vi "Receiver_Example - 2 Channel - Experiment_6.vi"() -> ()   [LabVIEW 2022 SP3]
panel:
  out "iterationsIM":dbl
  in  "State":i32
  in  "Counter":dbl
  in  "OFDM - 4QAM/16QAM":bool
  out "Iterations 2":i32
  in  "Tab Control 3":enum32{"OFDM - 4QAM", "16QAM"}(tab)
  in  "Tab Control":enum32{"USRP Parameters", "Rx Info", "BER"}(tab)
  in  "USRP ControledParameters":T1={"Active Antenna"="RX2", "Gain (dB)"=10.0, "Carrier Frequency"=2400000000.0, "IQ Rate"=2000000.0, "Active channels"="0,1"} {"IQ Rate" format="%#_6p"; "Carrier Frequency" format="%#_6p"; "Gain (dB)" format="%#_6f"}
  in  "Device selection":refnum<k15>="RIO0"
  in  "Trigger level":dbl=0.005 format="%f"
  out "CH0":T2
  out "CH1":T2
  out "SIG valid? - CH1":bool
  out "SIG valid? - CH0":bool
  out "Frequency offset - CH1":dbl
  out "Frequency offset - CH0":dbl
  out "Coerced Parameters":T3={"IQ Rate"=100000.0, "Carrier  Freq."=100000.0, "Gain"=0.0} {"Gain" format="%#_6f"; "Carrier  Freq." format="%#_6p"; "IQ Rate" format="%#_6p"}
  out "Error out":errorcluster
  in  "Expected message LP - CH0":string="Non Critical Data\nNon Critical Data\nNon Critical Data\nNon Critical Data\nNon Critical Data"
  in  "Expected message - CH1":string="Critical Dataaaaa\nCritical Dataaaaa\nCritical Dataaaaa\nCritical Dataaaaa\nCritical Dataaaaa"
  out "Expected message LP Detected CH0":string="Non Critical Data\nNon Critical Data\nNon Critical Data\nNon Critical Data\nNon Critical Data"
  out "Expected message HP Detected CH1":string="Non Critical Data\nNon Critical Data\nNon Critical Data\nNon Critical Data\nNon Critical Data"
  in  "Boolean":bool
  in  "Boolean 3":bool
  out "Expected message HP Detected CH0":string="Non Critical Data\nNon Critical Data\nNon Critical Data\nNon Critical Data\nNon Critical Data"
  in  "Expected message HP - CH0":string="Critical Dataaaaa\nCritical Dataaaaa\nCritical Dataaaaa\nCritical Dataaaaa\nCritical Dataaaaa"
  in  "Boolean 2":bool
  out "Inst. BER HP - CH0":dbl format="%#_4g"
  out "Acc. BER HP - CH0":dbl format="%#_4g"
  out "Acum. Err HP - CH0":dbl
  out "No. Bits HP - CH0":dbl
  out "Acc. BER LP - CH0":dbl format="%#_4g"
  out "Inst. BER - CH1":dbl format="%#_4g"
  out "Inst. BER LP - CH0":dbl format="%#_4g"
  out "No. Bits - CH1":dbl
  out "No. Bits LP - CH0":dbl
  out "Acum. Err - CH1":dbl
  out "Acum. Err LP - CH0":dbl
  in  "Record BER":bool
  in  "Refresh Button":bool
  out "Acc. BER - CH1":dbl format="%#_4g"
  in  "Low-Power Window Size - CH0":dbl=15.0 format="%#_6p"
  in  "High-Power Window Size":dbl=15.0 format="%#_6p"
  out "High-Power Image 2":T4(plugin-control)
  in  "Tab Control 2":enum32{"1 Channel", "2 Channel"}(tab)
  out "Constellation Map 1 Channel":cdb[](graph)
  out "Low-Power BER - 1 Channel":dbl(graph)
  out "High-Power BER - 1 Channel":dbl(graph)
  out "High-Power Decoded message - 1 Channel":string
  out "Low-Power Decoded message - 1 Channel":string
  out "Low-Power Decoded message - CH0":string
  out "Decoded message - CH1":string
  out "Constellation Map 2 Channel":cluster{"Constellation":cdb[]}[](graph)
  out "Low-Power BER - CH0":dbl(graph)
  out "High-Power BER":T5(graph)
  out "High-Power Decoded message - CH0":string
  out "CH1 2":bool
  out "CH0 2":bool
  in  "Channel":bool
  out "Reconstructed Image":T4(plugin-control)
  out "Expected message  HP  Detected 2":string="Critical Dataaaaa\nCritical Dataaaaa\nCritical Dataaaaa\nCritical Dataaaaa\nCritical Dataaaaa"
  in  "Boolean 4":bool
  in  "High-Power Window Size 2":dbl=15.0 format="%#_6p"
  out "High-Power Instantaneous BER Graph 2":u8(slide) scale=0.0..100.0
  out "High-Power BER Graph 2":dbl(graph)
  out "No. Bits HP 2":dbl
  out "Acc. BER  HP 2":dbl format="%#_4g"
  out "Acum. Err HP 2":dbl
  out "Inst. BER HP 2":dbl format="%#_4g"
  in  "Expected message 2 HP 2":string="Critical Dataaaaa\nCritical Dataaaaa\nCritical Dataaaaa\nCritical Dataaaaa\nCritical Dataaaaa"
  out "High-Power Decoded Message 2":string
  in  "Record BER 2":bool
  out "Constellation Map 2":cdb[](graph)
  out "Frequency offset 2":dbl
  out "SIG valid? 2":bool
  in  "Refresh Button 2":bool
  out "Error out 2":errorcluster
  in  "error in (no error)":errorcluster
  # "OFDM Superposition Coded Receiver"
  # "1 Channel"
  # "2 Channel"
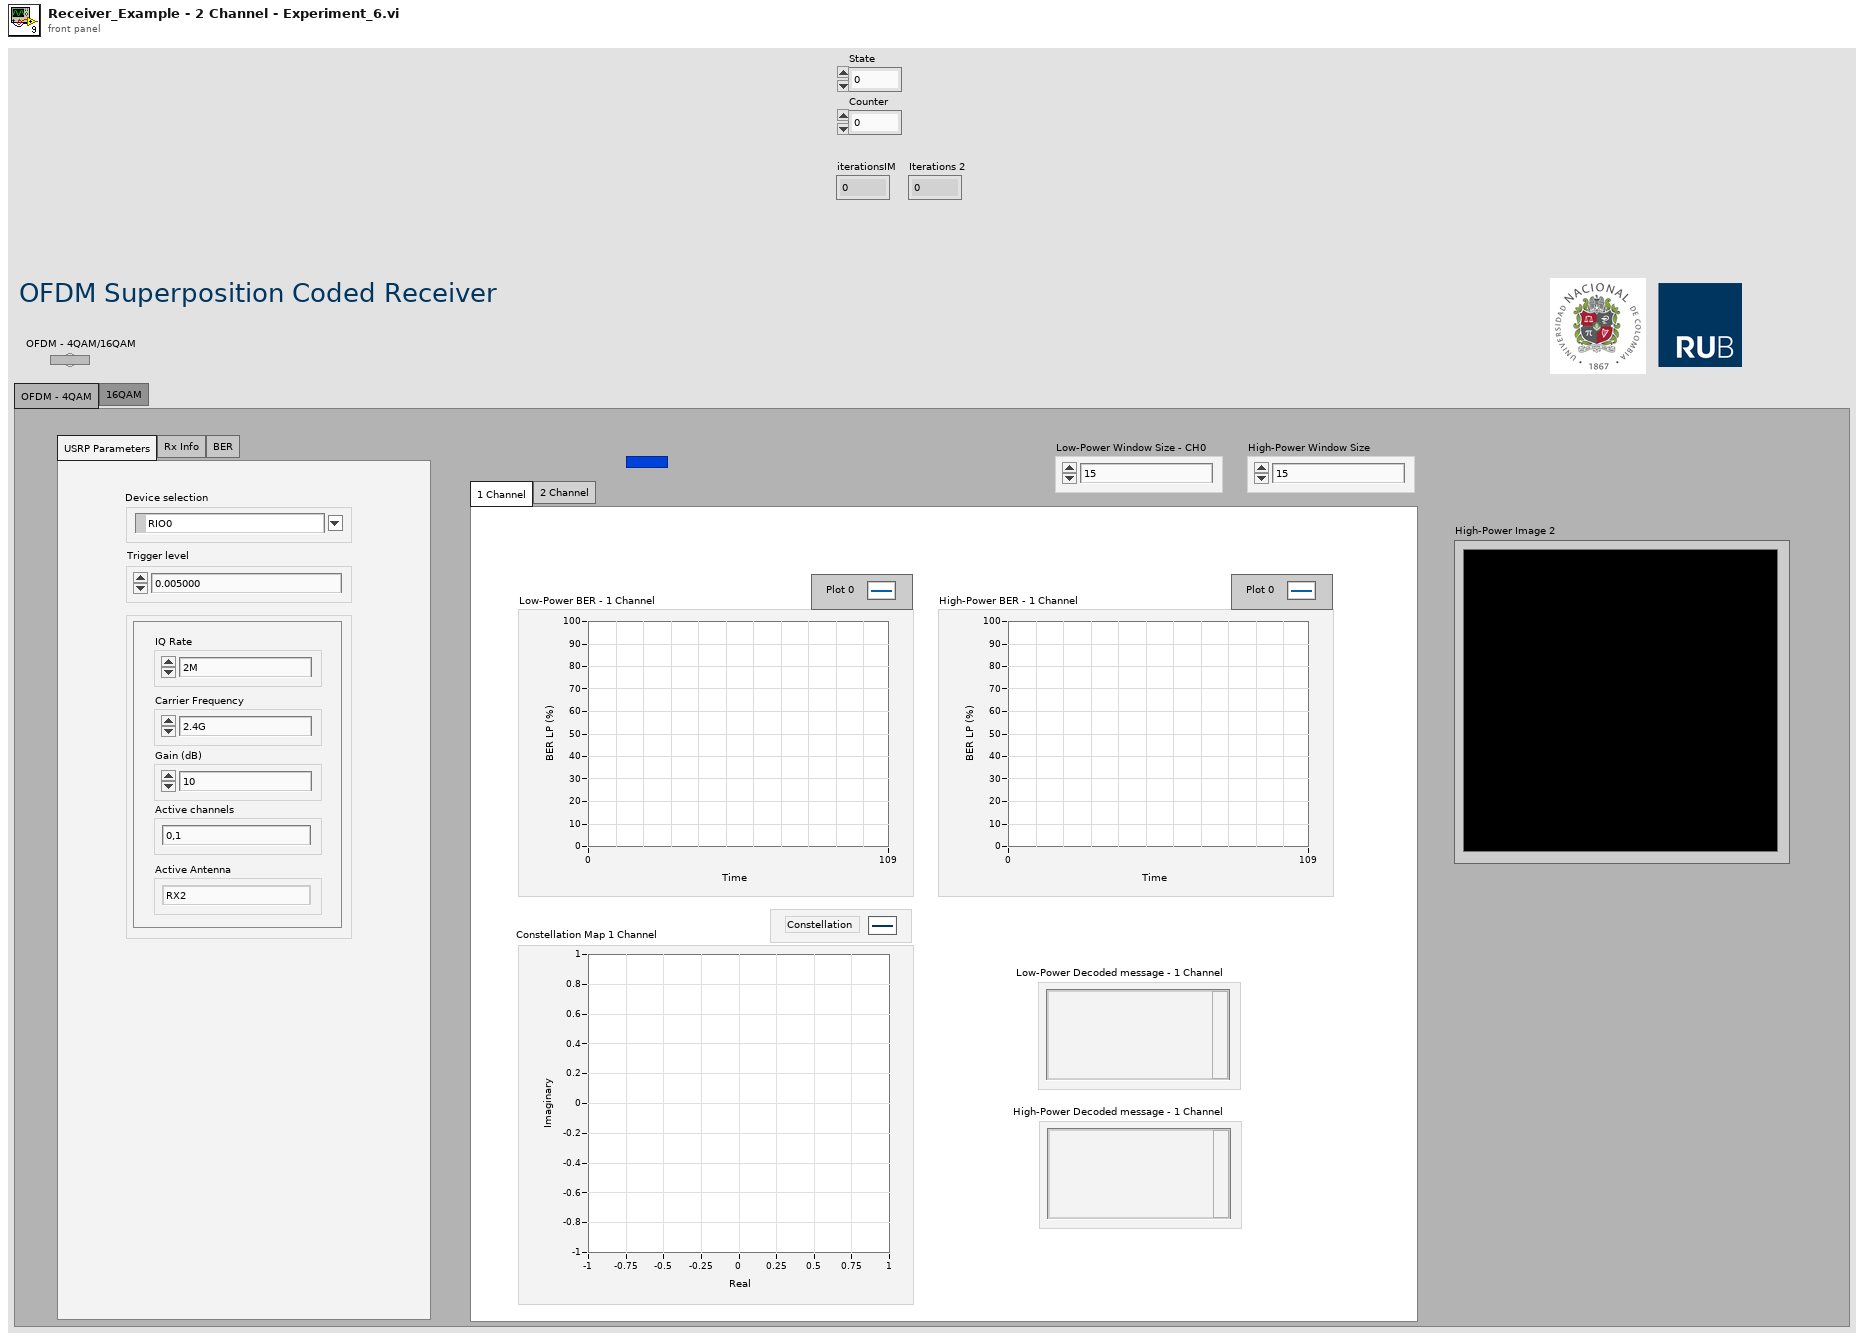
[diagram p1: front panel]
types:
  T1 = cluster{"Active Antenna":string, "Gain (dB)":dbl, "Carrier Frequency":dbl, "IQ Rate":dbl, "Active channels":string}
  T2 = cluster{"Modulation type":enum16{"QPSK(4QAM)", "64QAM", "16QAM", "BPSK"}, "BCC rate (k/n)":enum16{"1/2", "2/3", "3/4"}}
  T3 = cluster{"IQ Rate":dbl, "Carrier  Freq.":dbl, "Gain":dbl}
  T4 = typedef "IMAQ Image.ctl" = refnum<image>
  T5 = cluster{"Graph Instantaneous BER":dbl, "Graph Instantaneous BER":dbl, "Inst. BER - CH1":dbl}
  T6 = cluster{"coerced IQ rate":dbl, "coerced carrier frequency":dbl, "coerced gain":dbl}
  T7 = cluster{"Graph Instantaneous BER":dbl, "Graph Instantaneous BER":dbl, "Graph Instantaneous BER":dbl}
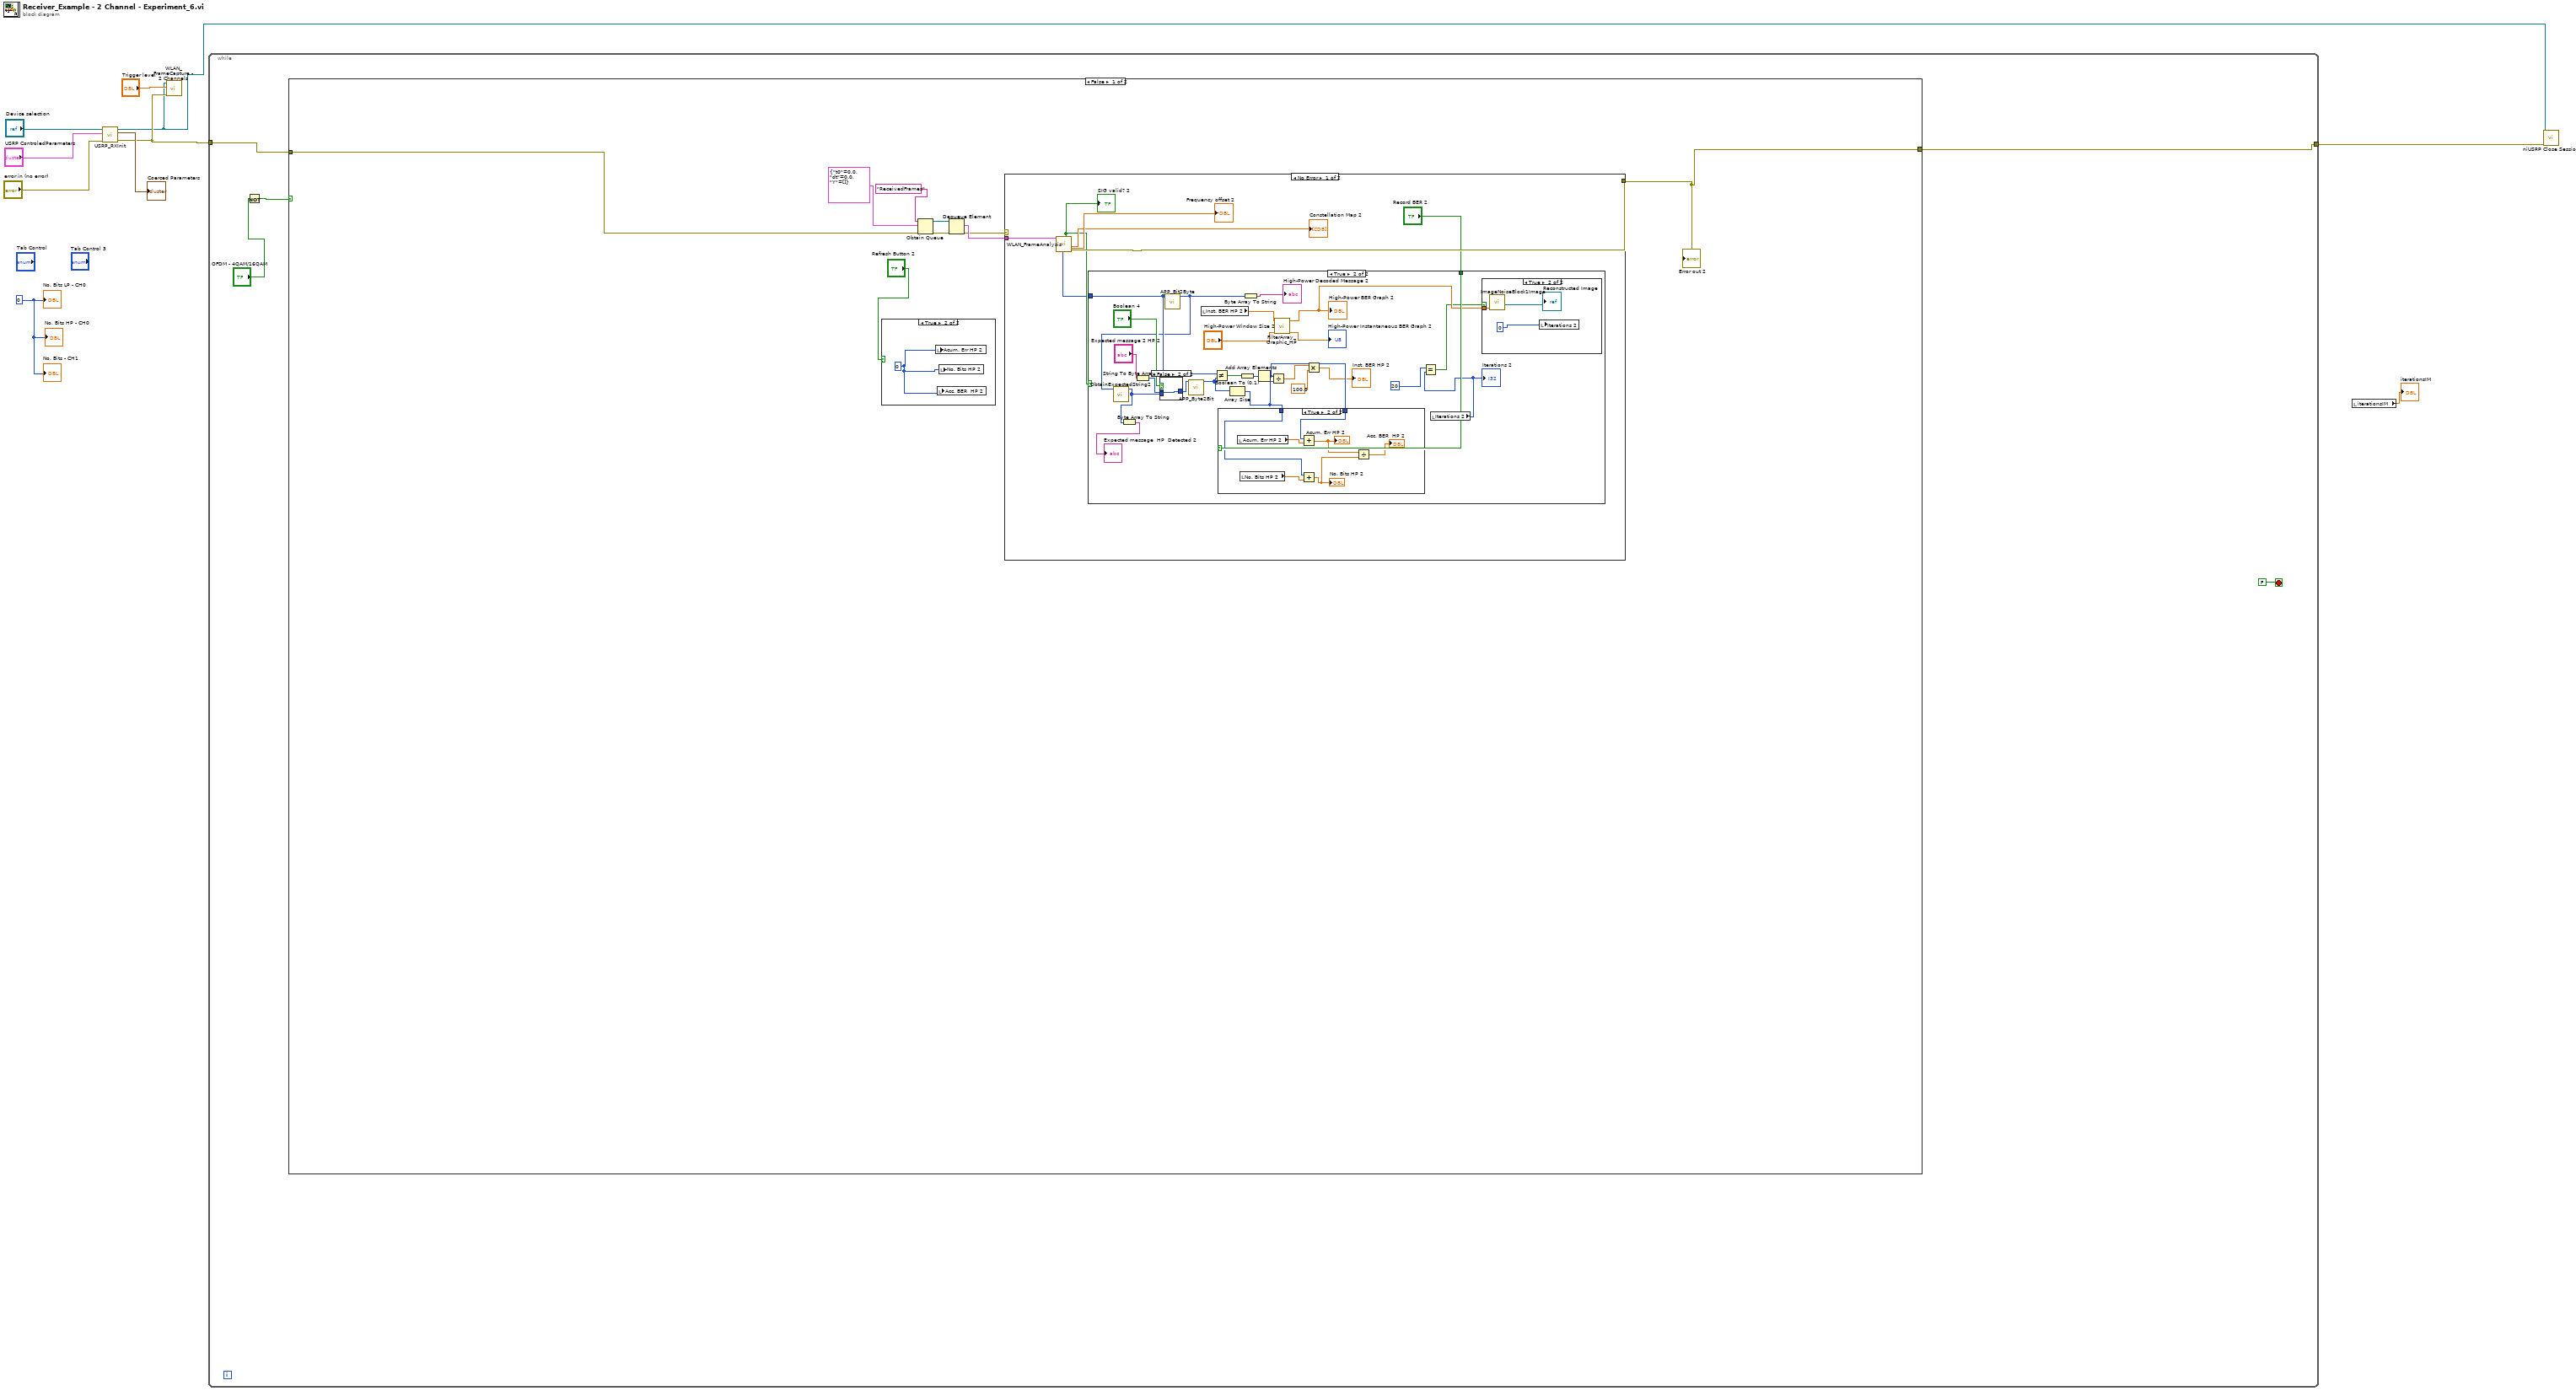
[diagram p0: block diagram]
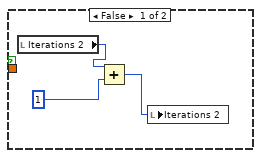
[diagram p4: hidden frame]
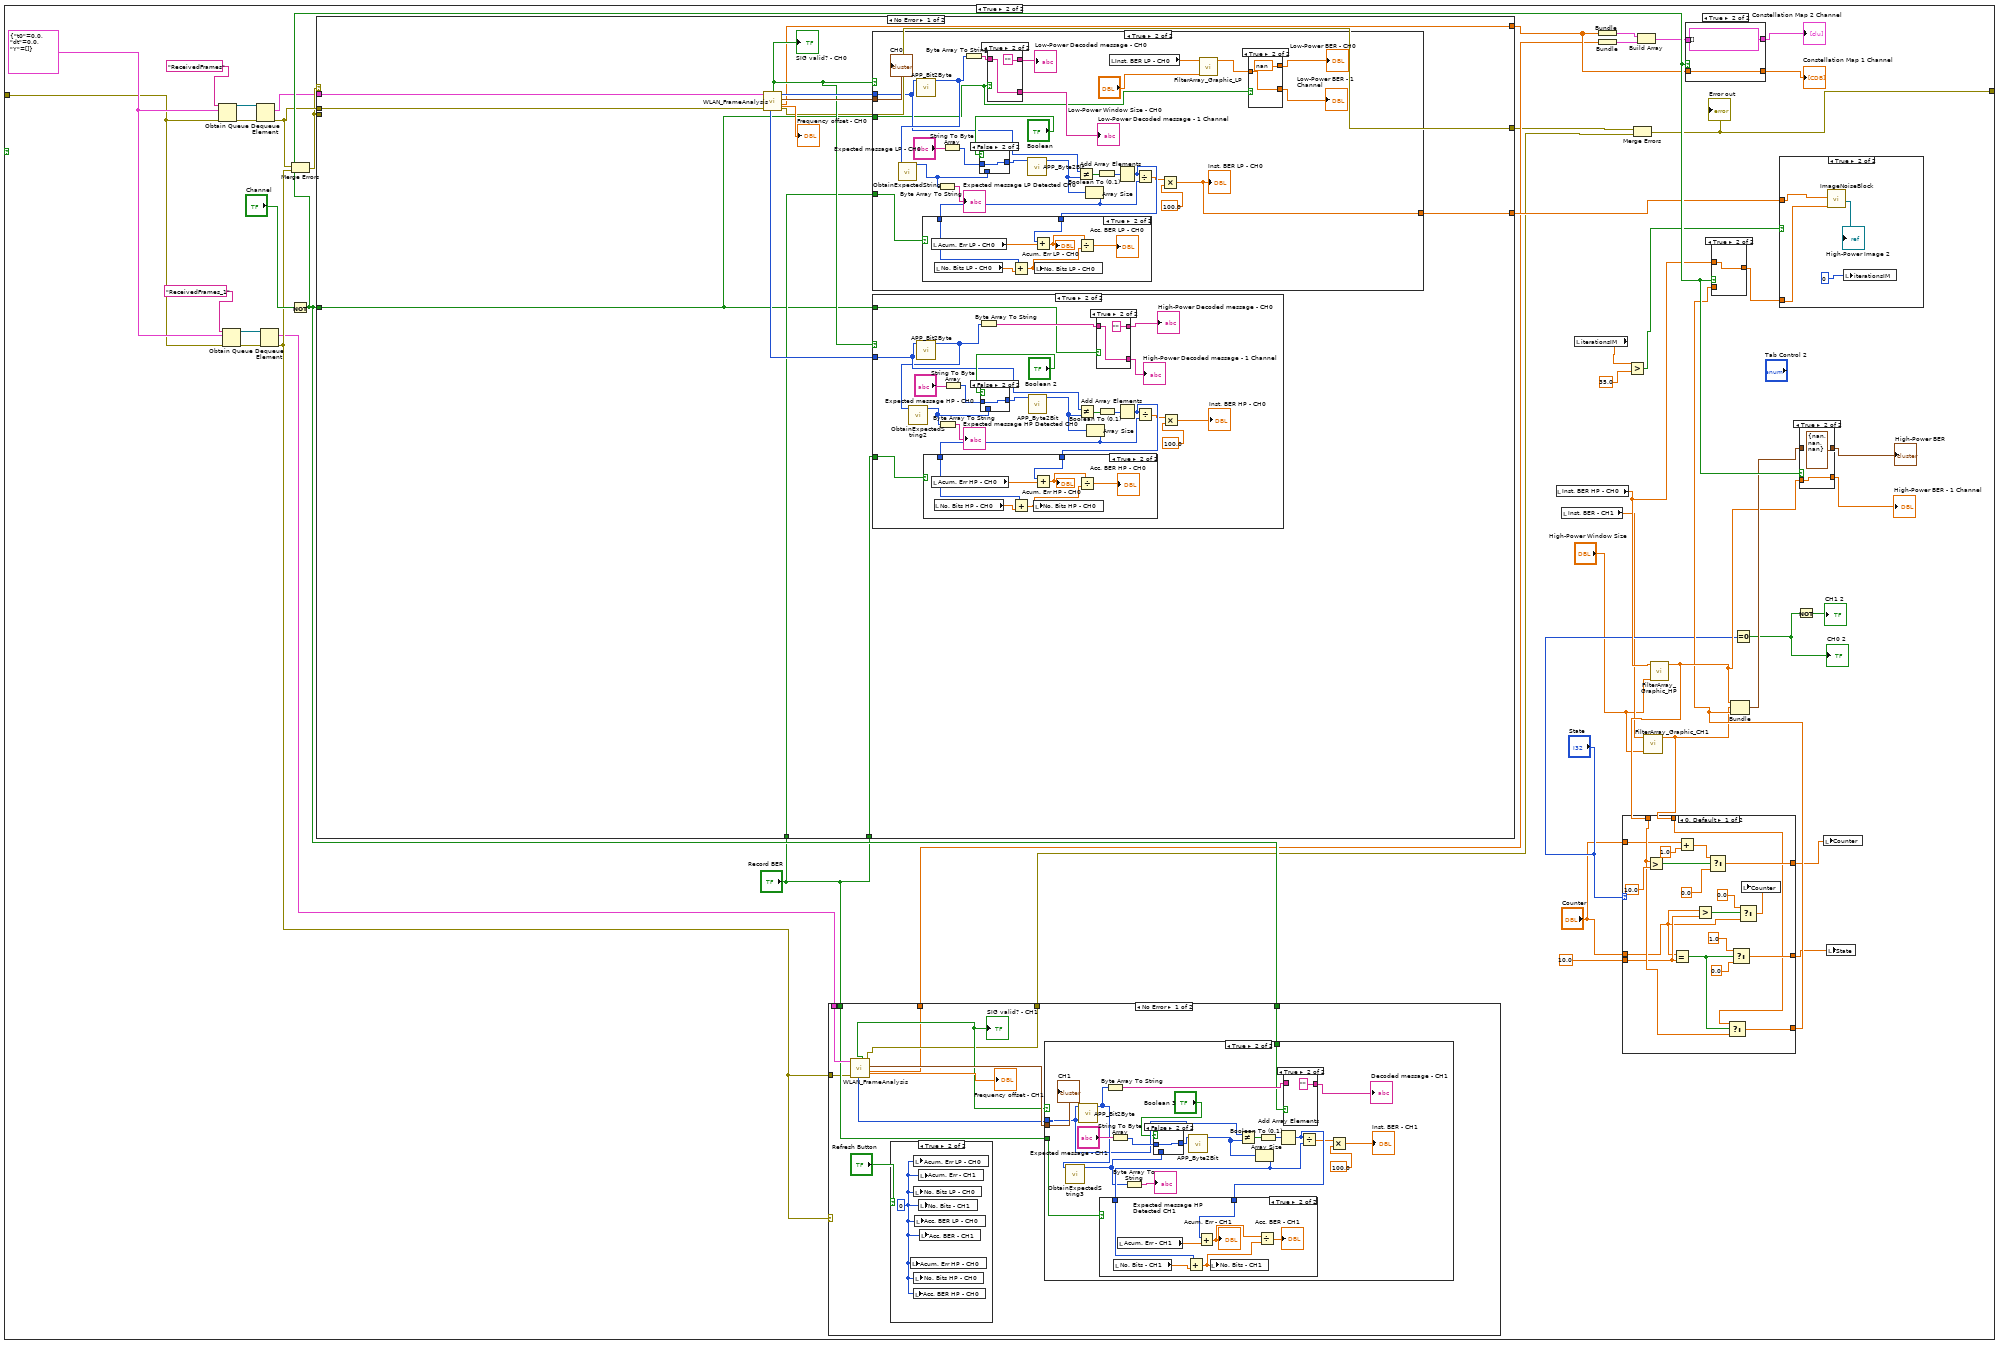
[diagram p8: hidden frame]
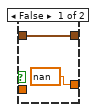
[diagram p9: hidden frame]
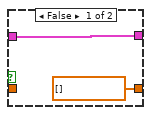
[diagram p11: hidden frame]
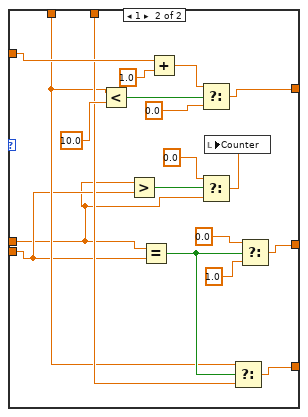
[diagram p12: hidden frame]
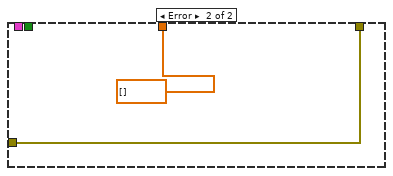
[diagram p18: hidden frame]
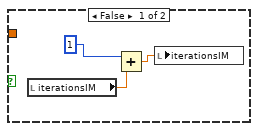
[diagram p19: hidden frame]
diagram:
  w2 = 0
  n1 = call "USRP_RXInit.vi"("device names"="Device selection", "USRP ControledParameters"="USRP ControledParameters", "error in (no error)"="error in (no error)") -> ("session handle out"=w5:refnum<k15>, "USRP CoercedParamters"=→"Coerced Parameters":T6, "error out"=w8:errorcluster)  [unwired: 5 in]
  n2 = call "WLAN_FrameCapture - 2 Channels.vi"("error in (no error)"=w8, "Trigger level"="Trigger level", "session handle"=w5) -> ()  [unwired: 8 in]
  n3 = while {
    tunnel: w8 -> [w15]
    tunnel: [w14] -> w6
    stop <- FALSE stop-if-true
    n4 = Not(x="OFDM - 4QAM/16QAM") -> (.not. x?=w12:bool)
    n5 = case shown="False" w12 {
      tunnel: w15 -> [w17 w75]
      tunnel: [w16 w74] -> w14
      frame False {
        n6 = case shown="True" "Refresh Button 2" {
          frame False {
          }
          frame True {
            w25 = 0
            n7 = local write "Acum. Err HP 2"(w25) -> ()
            n8 = local write "Acc. BER  HP 2"(w25) -> ()
            n9 = local write "No. Bits HP 2"(w25) -> ()
          }
        }
        n10 = Obtain Queue(name (unnamed)="ReceivedFrames", element data type=cluster{"t0":dbl, "dt":dbl, "Y":cdb[]} {"t0"=0.0, "dt"=0.0, "Y"=[]} ("data"), error in (no error)=w17) -> (queue out=w18:refnum<queue>, error out=w21:errorcluster)  [unwired: 2 in, 1 out]
        n11 = Dequeue Element(queue=w18, error in (no error)=w21) -> (element=w20:cluster{"t0":dbl, "dt":dbl, "Y":cdb[]}, error out=w19:errorcluster)  [unwired: 1 in, 2 out]
        n12 = case shown="No Error" w19 {
          selector: w19 -> [_ w73]
          tunnel: w20 -> [w31 _]
          tunnel: [w32 w73] -> w16
          frame No Error {
            n13 = call "WLAN_FrameAnalysis.vi"("input cluster"=w31) -> ("error out"=w32:errorcluster, "Constellation"=→"Constellation Map 2":cdb[], "Frequency offset"=→"Frequency offset 2":dbl, "SIG valid?"=w27:bool, "outputbitsHP"=w26:i8[])  [unwired: 4 in, 2 out]
            "SIG valid? 2" <- w27
            n14 = case shown="True" w27 {
              tunnel: "Record BER 2" -> [_ w51]
              tunnel: w26 -> [_ w46]
              frame False {
              }
              frame True {
                n15 = String To Byte Array(string="Expected message 2 HP 2") -> (unsigned byte array=w44:u8[])
                n16 = call "APP_Bit2Byte.vi"("input bit stream"=w46) -> ("output byte stream"=w40:u8[])  [unwired: 10 in]
                n17 = call "ObtainExpectedString2.vi"("Array"=w40) -> ("detectedMessage"=w42:i8[])  [unwired: 9 in]
                n18 = Byte Array To String(unsigned byte array=w42) -> (string=→"Expected message  HP  Detected 2":string)
                n19 = case shown="False" "Boolean 4" {
                  tunnel: [w64 w65] -> w45
                  tunnel: w44 -> [_ w65]
                  tunnel: w42 -> [w64 _]
                  frame True {
                  }
                  frame False {
                  }
                }
                n20 = call "APP_Byte2Bit.vi"("input byte stream"=w45) -> ("output bit stream"=w47:i8[])  [unwired: 10 in]
                n21 = local read "Inst. BER HP 2"() -> (w50:dbl)
                n22 = Not Equal?(x=w46, y=w47) -> (x != y?=w55:bool[])
                n23 = Array Size(array=w47) -> (size(s)=w52:i32)
                n24 = Boolean To (0,1)(Boolean=w55) -> (0, 1=w54:i16[])
                n25 = Byte Array To String(unsigned byte array=w40) -> (string=→"High-Power Decoded Message 2":string)
                n26 = Add Array Elements(numeric array=w54) -> (sum=w53:i16)
                n27 = case shown="True" w51 {
                  tunnel: w53 -> [_ w71]
                  tunnel: w52 -> [_ w66]
                  frame False {
                  }
                  frame True {
                    n28 = local read "Acum. Err HP 2"() -> (w72:dbl)
                    n29 = local read "No. Bits HP 2"() -> (w68:dbl)
                    n30 = Add(x=w71, y=w72) -> (x+y=w70:dbl)
                    "Acum. Err HP 2" <- w70
                    n31 = Add(x=w66, y=w68) -> (x+y=w67:dbl)
                    "No. Bits HP 2" <- w67
                    n32 = Divide(x=w70, y=w67) -> (x/y=→"Acc. BER  HP 2":dbl)
                  }
                }
                n33 = Divide(x=w53, y=w52) -> (x/y=w39:dbl)
                n34 = call "FilterArray_Graphic_HP.vi"("Window Size"="High-Power Window Size 2", "Instantaneous BER"=w50) -> ("Slide Bar"=→"High-Power Instantaneous BER Graph 2":dbl, "Graph Instantaneous BER"=w36:dbl)  [unwired: 4 in]
                "High-Power BER Graph 2" <- w36
                n35 = Multiply(x=w39, y=100.0) -> (x*y=→"Inst. BER HP 2":dbl)
                n36 = local read "Iterations 2"() -> (w34:i32)
                "Iterations 2" <- w34
                n37 = Equal?(x=20, y=w34) -> (x = y?=w33:bool)
                n38 = case shown="True" w33 {
                  tunnel: w36 -> [_ w63]
                  frame False {
                    n39 = local read "Iterations 2"() -> (w60:i32)
                    n40 = Add(x=w60, y=1) -> (x+y=w58:i32)
                    n41 = local write "Iterations 2"(w58) -> ()
                  }
                  frame True {
                    n42 = call "ImageNoiseBlock1Image.vi"("BERHP"=w63) -> ("High-Power Image"=→"Reconstructed Image":T4)  [unwired: 9 in]
                    n43 = local write "Iterations 2"(0) -> ()
                  }
                }
              }
            }
          }
          frame Error {
          }
        }
        "Error out 2" <- w16
      }
      frame True {
        w120 = cluster{"t0":dbl, "dt":dbl, "Y":cdb[]} {"t0"=0.0, "dt"=0.0, "Y"=[]} ("data")
        n44 = Obtain Queue(name (unnamed)="ReceivedFrames", element data type=w120, error in (no error)=w75) -> (queue out=w76:refnum<queue>, error out=w78:errorcluster)  [unwired: 2 in, 1 out]
        n45 = Obtain Queue(name (unnamed)="ReceivedFrames_1", element data type=w120, error in (no error)=w75) -> (queue out=w80:refnum<queue>, error out=w81:errorcluster)  [unwired: 2 in, 1 out]
        n46 = Dequeue Element(queue=w76, error in (no error)=w78) -> (element=w77:cluster{"t0":dbl, "dt":dbl, "Y":cdb[]}, error out=w84:errorcluster)  [unwired: 1 in, 2 out]
        n47 = Dequeue Element(queue=w80, error in (no error)=w81) -> (element=w89:cluster{"t0":dbl, "dt":dbl, "Y":cdb[]}, error out=w93:errorcluster)  [unwired: 1 in, 2 out]
        n48 = Not(x="Channel") -> (.not. x?=w119:bool)
        n49 = Merge Errors(w84, w93) -> (w83:errorcluster)
        n50 = case shown="No Error" w83 {
          tunnel: w77 -> [w231 _]
          tunnel: w83 -> [_ w315]
          tunnel: w84 -> [w228 _]
          tunnel: [w227 100] -> w95
          tunnel: [w226 dbl[] []] -> w107
          tunnel: [w225 w315] -> w90
          tunnel: "Record BER" -> [w224 _]
          tunnel: "Record BER" -> [w223 _]
          tunnel: w119 -> [w222 _]
          frame No Error {
            n51 = call "WLAN_FrameAnalysis.vi"("error in (no error)"=w228, "input cluster"=w231) -> ("error out"=w225:errorcluster, "Constellation"=w226:cdb[], "Modulation parameter"=w232:T2, "output bits"=w233:i8[], "Frequency offset"=→"Frequency offset - CH0":dbl, "SIG valid?"=w229:bool, "outputbitsHP"=w230:i8[])  [unwired: 3 in]
            "SIG valid? - CH0" <- w229
            n52 = case shown="True" w229 {
              tunnel: w233 -> [_ w278]
              tunnel: w232 -> [_ w296]
              tunnel: w223 -> [_ w292]
              tunnel: [100.0 w277] -> w227
              tunnel: w222 -> [_ w270]
              frame False {
              }
              frame True {
                n53 = call "APP_Bit2Byte.vi"("input bit stream"=w278) -> ("output byte stream"=w282:u8[])  [unwired: 10 in]
                n54 = call "ObtainExpectedString.vi"("Array"=w282) -> ("detectedMessage"=w279:i8[])  [unwired: 9 in]
                n55 = Byte Array To String(unsigned byte array=w279) -> (string=→"Expected message LP Detected CH0":string)
                n56 = String To Byte Array(string="Expected message LP - CH0") -> (unsigned byte array=w283:u8[])
                n57 = Byte Array To String(unsigned byte array=w282) -> (string=w276:string)
                n58 = case shown="False" "Boolean" {
                  tunnel: [w305 w306] -> w285
                  tunnel: w283 -> [_ w306]
                  tunnel: w279 -> [w305 _]
                  frame True {
                  }
                  frame False {
                  }
                }
                n59 = case shown="True" w270 {
                  tunnel: w276 -> [w302 w304]
                  tunnel: ["" ("string") w304] -> w275
                  tunnel: [w302 "" ("string")] -> w274
                  frame False {
                  }
                  frame True {
                  }
                }
                "Low-Power Decoded message - CH0" <- w274
                "Low-Power Decoded message - 1 Channel" <- w275
                n60 = call "APP_Byte2Bit.vi"("input byte stream"=w285) -> ("output bit stream"=w284:i8[])  [unwired: 10 in]
                n61 = Not Equal?(x=w278, y=w284) -> (x != y?=w294:bool[])
                n62 = Array Size(array=w284) -> (size(s)=w291:i32)
                n63 = Boolean To (0,1)(Boolean=w294) -> (0, 1=w295:i16[])
                n64 = local read "Inst. BER LP - CH0"() -> (w288:dbl)
                n65 = Add Array Elements(numeric array=w295) -> (sum=w290:i16)
                n66 = case shown="True" w292 {
                  tunnel: w291 -> [_ w312]
                  tunnel: w290 -> [_ w310]
                  frame False {
                  }
                  frame True {
                    n67 = local read "Acum. Err LP - CH0"() -> (w311:dbl)
                    n68 = local read "No. Bits LP - CH0"() -> (w313:dbl)
                    n69 = Add(x=w312, y=w313) -> (x+y=w309:dbl)
                    n70 = Add(x=w310, y=w311) -> (x+y=w308:dbl)
                    "Acum. Err LP - CH0" <- w308
                    n71 = local write "No. Bits LP - CH0"(w309) -> ()
                    n72 = Divide(x=w308, y=w309) -> (x/y=→"Acc. BER LP - CH0":dbl)
                  }
                }
                n73 = Divide(x=w290, y=w291) -> (x/y=w287:dbl)
                n74 = Multiply(x=w287, y=100.0) -> (x*y=w277:dbl)
                "Inst. BER LP - CH0" <- w277
                n75 = call "FilterArray_Graphic_LP.vi"("Window Size"="Low-Power Window Size - CH0", "Instantaneous BER"=w288) -> ("Graph Instantaneous BER"=w273:dbl)  [unwired: 4 in, 1 out]
                n76 = case shown="True" w270 {
                  tunnel: w273 -> [w298 w300]
                  tunnel: [nan ("Graph Instantaneous BER") w300] -> w272
                  tunnel: [w298 nan ("Graph Instantaneous BER")] -> w271
                  frame False {
                  }
                  frame True {
                  }
                }
                "Low-Power BER - CH0" <- w271
                "Low-Power BER - 1 Channel" <- w272
                "CH0" <- w296
              }
            }
            n77 = case shown="True" w229 {
              tunnel: w230 -> [_ w242]
              tunnel: w224 -> [_ w252]
              tunnel: w222 -> [_ w235]
              frame False {
              }
              frame True {
                n78 = call "APP_Bit2Byte.vi"("input bit stream"=w242) -> ("output byte stream"=w241:u8[])  [unwired: 10 in]
                n79 = call "ObtainExpectedString2.vi"("Array"=w241) -> ("detectedMessage"=w240:i8[])  [unwired: 9 in]
                n80 = Byte Array To String(unsigned byte array=w240) -> (string=→"Expected message HP Detected CH0":string)
                n81 = String To Byte Array(string="Expected message HP - CH0") -> (unsigned byte array=w245:u8[])
                n82 = Byte Array To String(unsigned byte array=w241) -> (string=w236:string)
                n83 = case shown="False" "Boolean 2" {
                  tunnel: [w260 w261] -> w247
                  tunnel: w245 -> [_ w261]
                  tunnel: w240 -> [w260 _]
                  frame True {
                  }
                  frame False {
                  }
                }
                n84 = call "APP_Byte2Bit.vi"("input byte stream"=w247) -> ("output bit stream"=w246:i8[])  [unwired: 10 in]
                n85 = Not Equal?(x=w242, y=w246) -> (x != y?=w254:bool[])
                n86 = Array Size(array=w246) -> (size(s)=w251:i32)
                n87 = case shown="True" w235 {
                  tunnel: w236 -> [w257 w259]
                  tunnel: ["" ("string") w259] -> w237
                  tunnel: [w257 "" ("string")] -> w238
                  frame False {
                  }
                  frame True {
                  }
                }
                "High-Power Decoded message - CH0" <- w238
                "High-Power Decoded message - 1 Channel" <- w237
                n88 = Boolean To (0,1)(Boolean=w254) -> (0, 1=w255:i16[])
                n89 = Add Array Elements(numeric array=w255) -> (sum=w250:i16)
                n90 = case shown="True" w252 {
                  tunnel: w251 -> [_ w267]
                  tunnel: w250 -> [_ w265]
                  frame False {
                  }
                  frame True {
                    n91 = local read "Acum. Err HP - CH0"() -> (w266:dbl)
                    n92 = local read "No. Bits HP - CH0"() -> (w268:dbl)
                    n93 = Add(x=w267, y=w268) -> (x+y=w264:dbl)
                    n94 = local write "No. Bits HP - CH0"(w264) -> ()
                    n95 = Add(x=w265, y=w266) -> (x+y=w263:dbl)
                    "Acum. Err HP - CH0" <- w263
                    n96 = Divide(x=w263, y=w264) -> (x/y=→"Acc. BER HP - CH0":dbl)
                  }
                }
                n97 = Divide(x=w250, y=w251) -> (x/y=w249:dbl)
                n98 = Multiply(x=w249, y=100.0) -> (x*y=→"Inst. BER HP - CH0":dbl)
              }
            }
          }
          frame Error {
            (unwired) 100
          }
        }
        n99 = case shown="No Error" w93 {
          tunnel: w89 -> [w175 _]
          tunnel: "Record BER" -> [w173 _]
          tunnel: [w172 w214] -> w91
          tunnel: [w171 dbl[] []] -> w92
          tunnel: w93 -> [w170 w214]
          tunnel: w119 -> [w169 _]
          frame No Error {
            n100 = call "WLAN_FrameAnalysis.vi"("error in (no error)"=w170, "input cluster"=w175) -> ("error out"=w172:errorcluster, "Constellation"=w171:cdb[], "Modulation parameter"=w178:T2, "Frequency offset"=→"Frequency offset - CH1":dbl, "SIG valid?"=w174:bool, "outputbitsHP"=w176:i8[])  [unwired: 3 in, 1 out]
            "SIG valid? - CH1" <- w174
            n101 = case shown="True" "Refresh Button" {
              frame False {
              }
              frame True {
                w180 = 0
                n102 = local write "Acum. Err HP - CH0"(w180) -> ()
                n103 = local write "Acc. BER HP - CH0"(w180) -> ()
                n104 = local write "Acum. Err LP - CH0"(w180) -> ()
                n105 = local write "No. Bits LP - CH0"(w180) -> ()
                n106 = local write "No. Bits HP - CH0"(w180) -> ()
                n107 = local write "Acc. BER LP - CH0"(w180) -> ()
                n108 = local write "Acum. Err - CH1"(w180) -> ()
                n109 = local write "No. Bits - CH1"(w180) -> ()
                n110 = local write "Acc. BER - CH1"(w180) -> ()
              }
            }
            n111 = case shown="True" w174 {
              tunnel: w176 -> [_ w187]
              tunnel: w178 -> [_ w201]
              tunnel: w173 -> [_ w184]
              tunnel: w169 -> [_ w181]
              frame False {
              }
              frame True {
                n112 = call "APP_Bit2Byte.vi"("input bit stream"=w187) -> ("output byte stream"=w190:u8[])  [unwired: 10 in]
                n113 = call "ObtainExpectedString3.vi"("Array"=w190) -> ("detectedMessage"=w189:i8[])  [unwired: 9 in]
                n114 = Byte Array To String(unsigned byte array=w190) -> (string=w182:string)
                n115 = String To Byte Array(string="Expected message - CH1") -> (unsigned byte array=w191:u8[])
                n116 = Byte Array To String(unsigned byte array=w189) -> (string=→"Expected message HP Detected CH1":string)
                n117 = case shown="False" "Boolean 3" {
                  tunnel: [w204 w205] -> w193
                  tunnel: w191 -> [_ w205]
                  tunnel: w189 -> [w204 _]
                  frame True {
                  }
                  frame False {
                  }
                }
                n118 = call "APP_Byte2Bit.vi"("input byte stream"=w193) -> ("output bit stream"=w192:i8[])  [unwired: 10 in]
                n119 = Not Equal?(x=w187, y=w192) -> (x != y?=w199:bool[])
                n120 = Array Size(array=w192) -> (size(s)=w197:i32)
                n121 = Boolean To (0,1)(Boolean=w199) -> (0, 1=w200:i16[])
                n122 = Add Array Elements(numeric array=w200) -> (sum=w196:i16)
                n123 = case shown="True" w184 {
                  tunnel: w197 -> [_ w211]
                  tunnel: w196 -> [_ w209]
                  frame False {
                  }
                  frame True {
                    n124 = local read "No. Bits - CH1"() -> (w212:dbl)
                    n125 = local read "Acum. Err - CH1"() -> (w210:dbl)
                    n126 = Add(x=w211, y=w212) -> (x+y=w208:dbl)
                    n127 = Add(x=w209, y=w210) -> (x+y=w207:dbl)
                    "Acum. Err - CH1" <- w207
                    n128 = local write "No. Bits - CH1"(w208) -> ()
                    n129 = Divide(x=w207, y=w208) -> (x/y=→"Acc. BER - CH1":dbl)
                  }
                }
                n130 = case shown="True" w181 {
                  tunnel: w182 -> [w202 _]
                  tunnel: [w202 "" ("string")] -> w183
                  frame False {
                  }
                  frame True {
                  }
                }
                "Decoded message - CH1" <- w183
                n131 = Divide(x=w196, y=w197) -> (x/y=w194:dbl)
                n132 = Multiply(x=w194, y=100.0) -> (x*y=→"Inst. BER - CH1":dbl)
                "CH1" <- w201
              }
            }
          }
          frame Error {
          }
        }
        n133 = local read "Inst. BER HP - CH0"() -> (w112:dbl)
        n134 = local read "Inst. BER - CH1"() -> (w101:dbl)
        n135 = local read "iterationsIM"() -> (w85:dbl)
        n136 = Bundle("Constellation"=w107) -> (w106:cluster{"Constellation":cdb[]})  [unwired: 1 in]
        n137 = Bundle("Constellation"=w92) -> (w88:cluster{"Constellation":cdb[]})  [unwired: 1 in]
        n138 = Greater?(x=w85, y=35.0) -> (0:w86:bool)
        n139 = Merge Errors(w90, w91) -> (w74:errorcluster)
        "Error out" <- w74
        n140 = Build Array(w106, w88) -> (w109:cluster{"Constellation":cdb[]}[])
        n141 = call "FilterArray_Graphic_CH1.vi"("Window Size"="High-Power Window Size", "Instantaneous BER"=w101) -> ("Graph Instantaneous BER"=w102:dbl)  [unwired: 4 in, 1 out]
        n142 = call "FilterArray_Graphic_HP.vi"("Window Size"="High-Power Window Size", "Instantaneous BER"=w112) -> ("Graph Instantaneous BER"=w115:dbl)  [unwired: 4 in, 1 out]
        n143 = case shown="0, Default" "State" {
          tunnel: "Counter" -> [w137 w157]
          tunnel: [w144 w160] -> w97
          tunnel: "Counter" -> [w132 w150]
          tunnel: [w141 w159] -> w98
          tunnel: [w139 w158] -> w114
          tunnel: w115 -> [w138 w155]
          tunnel: w102 -> [w136 w156]
          tunnel: 10.0 ("y") -> [w135 w151]
          frame 0, Default {
            n144 = Greater?(x=w138, y=10.0) -> (0:w145:bool)
            n145 = Equal?(x=w132, y=w135) -> (x = y?=w140:bool)
            n146 = Add(x=w137, y=1.0) -> (x+y=w147:dbl)
            n147 = Greater?(x=w132, y=w135) -> (0:w134:bool)
            n148 = Select(t=w147, s=w145, f=0.0) -> (s? t:f=w144:dbl)
            n149 = Select(t=w136, s=w140, f=w138) -> (s? t:f=w139:dbl)
            n150 = Select(t=1.0, s=w140, f=0.0) -> (s? t:f=w141:dbl)
            n151 = Select(t=0.0, s=w134, f=w132) -> (s? t:f=w131:dbl)
            n152 = local write "Counter"(w131) -> ()
          }
          frame 1 {
            n153 = Less?(x=w155, y=10.0) -> (x < y?=w161:bool)
            n154 = Greater?(x=w150, y=w151) -> (0:w153:bool)
            n155 = Equal?(x=w150, y=w151) -> (x = y?=w163:bool)
            n156 = Add(x=w157, y=1.0) -> (x+y=w167:dbl)
            n157 = Select(t=w167, s=w161, f=0.0) -> (s? t:f=w160:dbl)
            n158 = Select(t=0.0, s=w153, f=w150) -> (s? t:f=w154:dbl)
            n159 = local write "Counter"(w154) -> ()
            n160 = Select(t=w155, s=w163, f=w156) -> (s? t:f=w158:dbl)
            n161 = Select(t=0.0, s=w163, f=1.0) -> (s? t:f=w159:dbl)
          }
        }
        n162 = case shown="True" w119 {
          tunnel: [cdb[] [] ("Constellation") w130] -> w108
          tunnel: w107 -> [_ w130]
          tunnel: w109 -> [w128 _]
          tunnel: [w128 cluster{"Constellation":cdb[]}[] []] -> w110
          frame False {
          }
          frame True {
          }
        }
        "Constellation Map 2 Channel" <- w110
        "Constellation Map 1 Channel" <- w108
        n163 = case shown="True" w119 {
          tunnel: w112 -> [_ w126]
          tunnel: [w125 w126] -> w113
          tunnel: w114 -> [w125 _]
          frame False {
          }
          frame True {
          }
        }
        n164 = Bundle("Graph Instantaneous BER"=w115, "Graph Instantaneous BER"=w102, "Graph Instantaneous BER"=w114) -> (w117:T7)  [unwired: 1 in]
        n165 = Equal To 0?(x="State") -> (x = 0?=w105:bool)
        "CH0 2" <- w105
        n166 = case shown="True" w86 {
          tunnel: w113 -> [_ w221]
          tunnel: w95 -> [_ w218]
          frame False {
            n167 = local read "iterationsIM"() -> (w217:dbl)
            n168 = Add(x=1, y=w217) -> (x+y=w216:dbl)
            n169 = local write "iterationsIM"(w216) -> ()
          }
          frame True {
            n170 = call "ImageNoiseBlock.vi"("BERLP"=w218, "BERHP"=w221) -> ("High-Power Image"=→"High-Power Image 2":T4)  [unwired: 8 in]
            n171 = local write "iterationsIM"(0) -> ()
          }
        }
        n172 = Not(x=w105) -> (.not. x?=→"CH1 2":bool)
        n173 = case shown="True" w119 {
          tunnel: w115 -> [_ w124]
          tunnel: [nan w124] -> w116
          tunnel: w117 -> [w122 _]
          tunnel: [w122 T7 {"Graph Instantaneous BER"=nan, "Graph Instantaneous BER"=nan, "Graph Instantaneous BER"=nan}] -> w118
          frame False {
          }
          frame True {
          }
        }
        "High-Power BER" <- w118
        "High-Power BER - 1 Channel" <- w116
        n174 = local write "Counter"(w97) -> ()
        n175 = local write "State"(w98) -> ()
      }
    }
  }
  n176 = local read "iterationsIM"() -> (→"iterationsIM":dbl)
  n177 = call <instrlib>:"niUSRP Close Session.vi"("session handle"=w5, "error in (no error)"=w6) -> ()  [unwired: 13 in, 1 out]
  "No. Bits LP - CH0" <- w2
  "No. Bits - CH1" <- w2
  "No. Bits HP - CH0" <- w2
